vi "GetAllTrianglesInfo.vi"() -> (2 "AllTriangles":T1[](array[typedef]), 3 "TriangleInfo":T3)   [LabVIEW 2014]
uses:
  TypeDefs/TriangleFace.ctl
  TypeDefs/Point3D.ctl
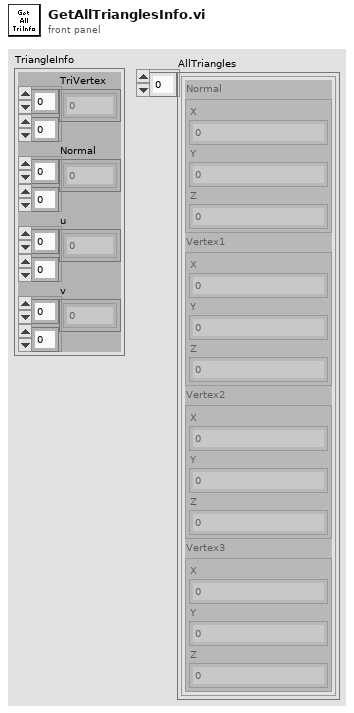
[diagram p1: front panel]
types:
  T1 = typedef "TriangleFace.ctl" = cluster{"Normal":T2, "Vertex1":T2, "Vertex2":T2, "Vertex3":T2}
  T2 = typedef "Point3D.ctl" = cluster{"X":sgl, "Y":sgl, "Z":sgl}
  T3 = cluster{"TriVertex":dbl[][], "Normal":dbl[][], "u":dbl[][], "v":dbl[][]}
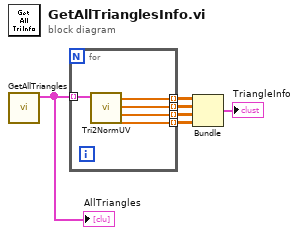
[diagram p0: block diagram]
diagram:
  n1 = call "GetAllTriangles.vi"() -> ("AllTriangles"=w6:T1[])  [unwired: 11 in]
  "AllTriangles" <- w6
  n2 = for {
    tunnel: w6 -> [w11] mode=indexing
    tunnel: [w10] -> w5 mode=indexing
    tunnel: [w9] -> w4 mode=indexing
    tunnel: [w8] -> w3 mode=indexing
    tunnel: [w7] -> w2 mode=indexing
    n3 = call "Tri2NormUV.vi"("TriangleFace"=w11) -> ("v"=w7:dbl[], "u"=w8:dbl[], "Normal"=w9:dbl[], "TriVertex"=w10:dbl[])  [unwired: 7 in]
  }
  n4 = Bundle("TriVertex"=w5, "Normal"=w4, "u"=w3, "v"=w2) -> (→"TriangleInfo":T3)  [unwired: 1 in]
